vi "DuplicateNode.vi"(7 "same parent?":bool, 8 "error in":errorcluster, 10 "new parent":T1, 11 "node ref in":T1) -> (0 "error out":errorcluster, 3 "new node ref":T1)   [LabVIEW 2025, in "CEF.lvlib"]
doc: "This VI duplicates a creates duplicate of a node.\nIf same parent is set to true the new node will use current parent, if set to false it will be added to the parent specified in the new parent terminalCopyright 2017 National Instruments Corporation\n\nLicensed under the Apache License, Version 2.0 (the \"License\"); you may not use this file except in compliance with the License. You may obtain a copy of the License at http://www.apache.org/licenses/LICENSE-2.0\nUnless required by applicable law or agreed to in writing, software distributed under the License is distributed on an \"AS IS\" BASIS, WITHOUT WARRANTIES OR CONDITIONS OF ANY KIND, either express or implied. See the License for the specific language governing permissions and limitations under the License."
uses:
  CEF.lvlib
  Node/NodeRef.ctl
  Node/CEF_Node.lvclass
  Node/CEF_Node.lvclass/CEF_Node.ctl
  Node/ReadParent.vi
  Node/ReadChildren.vi
  Node/WriteChildren.vi
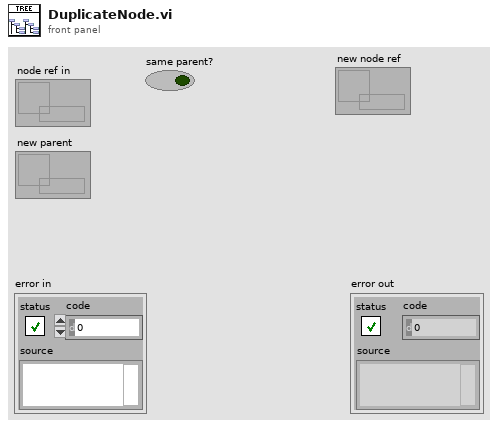
[diagram p1: front panel]
types:
  T1 = typedef "CEF.lvlib/CEF_Node.lvclass/NodeRef.ctl" = refnum<data-value>
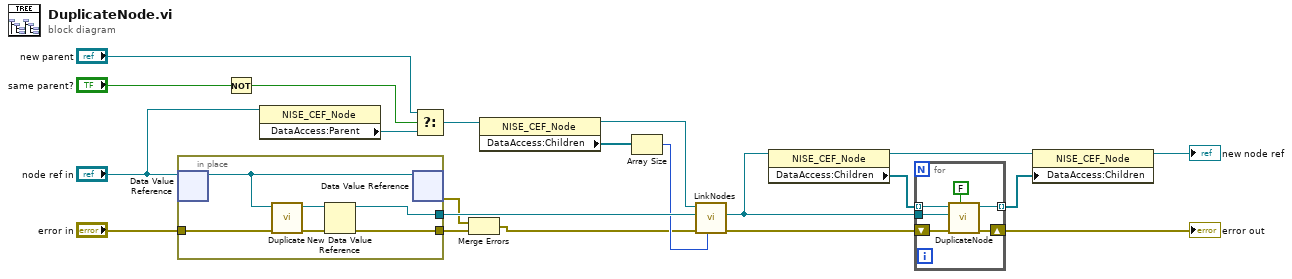
[diagram p0: block diagram]
diagram:
  n1 = in-place {
    in-place-border: [w27] -> w15
    in-place-border: "error in" -> [w25]
    in-place-border: [w23] -> w5
    n2 = in-place-dvr #1("node ref in") -> (w22:refnum<class "CEF_Node.lvclass">)  [unwired: 1 out]
    n3 = call-dynamic "Duplicate.vi"("error in"=w25, "node in"=w22) -> ("error out"=w24:errorcluster, "node copy out"=w26:refnum<class "CEF_Node.lvclass">)  [unwired: 8 in]
    n4 = New Data Value Reference(data value=w26, error in=w24) -> (data value reference=w27:refnum<data-value>, error out=w23:errorcluster)
    n5 = in-place-dvr #1(w22) -> (w6:errorcluster)  [unwired: 1 out]
  }
  n6 = Not(x="same parent?") -> (.not. x?=w3:bool)
  n7 = property class="NISE_CEF_Node"(reference="node ref in") -> ("DataAccess:Parent"=w2:T1)  [unwired: 1 in, 2 out]
  n8 = Select(t="new parent", s=w3, f=w2) -> (s? t:f=w10:T1)
  n9 = Merge Errors(w6, w5) -> (w4:errorcluster)
  n10 = property class="NISE_CEF_Node"(reference=w10) -> (reference out=w9:T1, "DataAccess:Children"=w8:T1[])  [unwired: 1 in, 1 out]
  n11 = Array Size(array=w8) -> (size(s)=w7:i32)
  n12 = call "LinkNodes.vi"("index"=w7, "error in"=w4, "child in"=w15, "parent in"=w9) -> ("error out"=w16:errorcluster, "child out"=w11:T1)  [unwired: 5 in, 1 out]
  n13 = property class="NISE_CEF_Node"(reference=w11) -> (reference out=w14:T1, "DataAccess:Children"=w13:T1[])  [unwired: 1 in, 1 out]
  n14 = for {
    tunnel: w13 -> [w33] mode=indexing
    tunnel: [w32] -> w12 mode=indexing
    tunnel: w11 -> [w31]
    shift-right: [w29] -> w20
    shift-left: w16 -> [w30]
    n15 = call "DuplicateNode.vi"("same parent?"=FALSE ("s"), "error in"=w30, "new parent"=w31, "node ref in"=w33) -> ("error out"=w29:errorcluster, "new node ref"=w32:T1)  [unwired: 6 in]
  }
  "error out" <- w20
  n16 = property class="NISE_CEF_Node"(reference=w14, "DataAccess:Children"=w12) -> (reference out=→"new node ref":T1)  [unwired: 1 in, 1 out]
